vi "Sorted Particle Report 2016.vi"(2 "Min Area Size %":dbl, 3 "Particle Count Limit":dbl=inf, 4 "Pixel Measurements":T1[](array[typedef])=[35, 4, 5, 6, 7] items=["Center of Mass X", "Center of Mass Y", "First Pixel X", "First Pixel Y", "Bounding Rect Left", "Bounding Rect Top", "Bounding Rect Right", "Bounding Rect Bottom", "Max Feret Diameter Start X", "Max Feret Diameter Start Y", "Max Feret Diameter End X", "Max Feret Diameter End Y", "Max Horiz. Segment Length Left", "Max Horiz. Segment Length Right", "Max Horiz. Segment Length Row", "-", "Bounding Rect Width", "Bounding Rect Height", "Bounding Rect Diagonal", "Perimeter", "Convex Hull Perimeter", "Holes' Perimeter", "Max Feret Diameter", "Equivalent Ellipse Major Axis", "Equivalent Ellipse Minor Axis", "Equivalent Ellipse Minor Axis (Feret)", "Equivalent Rect Long Side", "Equivalent Rect Short Side", "Equivalent Rect Diagonal", "Equivalent Rect Short Side (Feret)", "Average Horiz. Segment Length", "Average Vert. Segment Length", "Hydraulic Radius", "Waddel Disk Diameter", "-", "Area", "Holes' Area", "Particle & Holes' Area", "Convex Hull Area", "Image Area", "-", "Number of Holes", "Number of Horiz. Segments", "Number of Vert. Segments", "-", "Orientation", "Max Feret Diameter Orientation", "-", "% Area/Image Area", "% Area/(Particle & Holes' Area)", "Ratio of Equivalent Ellipse Axes", "Ratio of Equivalent Rect Sides", "-", "Elongation Factor", "Compactness Factor", "Heywood Circularity Factor", "Type Factor", "-", "Sum X", "Sum Y", "Sum XX", "Sum XY", "Sum YY", "Sum XXX", "Sum XXY", "Sum XYY", "Sum YYY", "-", "Moment of Inertia XX", "Moment of Inertia XY", "Moment of Inertia YY", "Moment of Inertia XXX", "Moment of Inertia XXY", "Moment of Inertia XYY", "Moment of Inertia YYY", "Norm. Moment of Inertia XX", "Norm. Moment of Inertia XY", "Norm. Moment of Inertia YY", "Norm. Moment of Inertia XXX", "Norm. Moment of Inertia XXY", "Norm. Moment of Inertia XYY", "Norm. Moment of Inertia YYY", "Hu Moment 1", "Hu Moment 2", "Hu Moment 3", "Hu Moment 4", "Hu Moment 5", "Hu Moment 6", "Hu Moment 7"], 5 "Image in":T2) -> (0 "Sorted Data":dbl[][](array[numeric]), 1 "Particles":i32)   [LabVIEW 2016]
doc: "Returns the requested measurements of a binary image sorted by the first parameter (often size), and limiting the rows in the 2D array by count and by size. Pass infinity to count to avoid a limit. Pass zero to size to avoid a limit."
uses:
  <vilib>/vision/Image Controls.llb/IMAQ Image.ctl
  <vilib>/vision/NI_Vision_Development_Module.lvlib
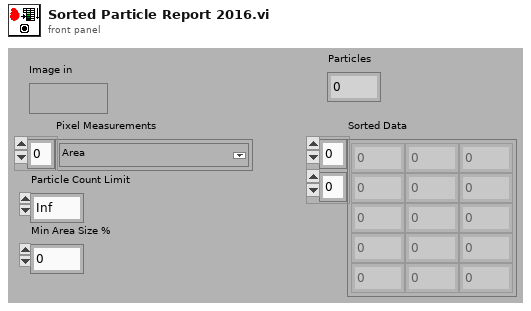
[diagram p1: front panel]
types:
  T1 = typedef "Particle Parameters" = i32
  T2 = typedef "IMAQ Image.ctl" = refnum<image>
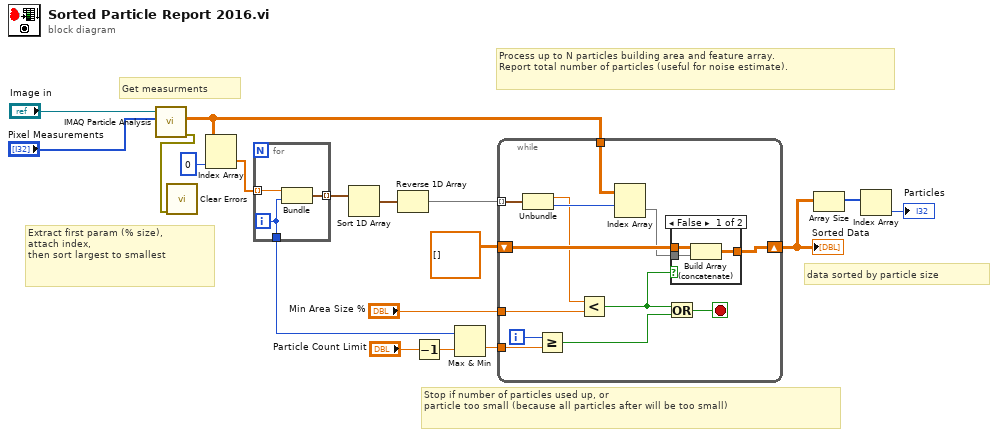
[diagram p0: block diagram]
diagram:
  # "data sorted by particle size"
  # "Stop if number of particles used up, or \nparticle too small (because all particles after will be too small)"
  # "Get measurments"
  # "Process up to N particles building area and feature array.\nReport total number of particles (useful for noise estimate)."
  # "Extract first param (% size), \nattach index, \nthen sort largest to smallest"
  n1 = call "IMAQ Particle Analysis"("Pixel Measurements"="Pixel Measurements", "Image"="Image in") -> ("error out"=w1:errorcluster, "Particle Measurements (Pixels)"=w12:dbl[][])  [unwired: 3 in, 5 out]
  n2 = call <vilib>:"Clear Errors.vi"("error in (no error)"=w1) -> ()  [unwired: 5 in, 2 out]
  n3 = Index Array(array=w12, index (col)=0 ("disabled index (col)")) -> (element=w15:dbl[])  [unwired: 1 in]
  n4 = for {
    tunnel: w15 -> [w21] mode=indexing
    tunnel: [w20] -> w16 mode=indexing
    tunnel: [w19] -> w2
    i -> [w19]
    n5 = Bundle("Numeric"=w21, w19) -> (w20:cluster{"Numeric":dbl, i32})  [unwired: 1 out]
  }
  n6 = Sort 1D Array(array=w16) -> (sorted array=w17:cluster{"Numeric":dbl, i32}[])
  n7 = Reverse 1D Array(array=w17) -> (reversed array=w5:cluster{"Numeric":dbl, i32}[])
  n8 = Decrement(x="Particle Count Limit") -> (x-1=w3:dbl)
  n9 = Max & Min(x=w2, y=w3) -> (min(x,y)=w4:dbl)  [unwired: 1 out]
  n10 = while {
    tunnel: w12 -> [w33]
    tunnel: w5 -> [w32] mode=indexing
    shift-right: [w29] -> w8
    shift-left: dbl[][] [] -> [w31]
    tunnel: w4 -> [w27]
    tunnel: "Min Area Size %" -> [w25]
    i -> [w28]
    stop <- w22 stop-if-true
    n11 = Unbundle(w32) -> ("Numeric"=w26:dbl, w34:i32)
    n12 = Greater Or Equal?(x=w28, y=w27) -> (x >= y?=w23:bool)
    n13 = Less?(x=w26, y=w25) -> (x < y?=w24:bool)
    n14 = Index Array(array=w33, index (row)=w34) -> (element=w30:dbl[])  [unwired: 1 in]
    n15 = Or(x=w24, y=w23) -> (x .or. y?=w22:bool)
    n16 = case shown="False" w24 {
      tunnel: w31 -> [w37 w38]
      tunnel: w30 -> [w36 _]
      tunnel: [w35 w38] -> w29
      frame False {
        n17 = Build Array (concatenate)(w37, w36) -> (w35:dbl[][])
      }
      frame True {
      }
    }
  }
  "Sorted Data" <- w8
  n18 = Array Size(array=w8) -> (size(s)=w7:i32[])
  n19 = Index Array(array=w7) -> (element=→"Particles":i32)  [unwired: 1 in]
